vi "RelaySwitcherB2023.vi"(8 "error in (no error)":errorcluster, 10 "RF Position":u16=1 min=1 max=63 step=1, 11 "Device In":cluster{"GPIB":u8, "Address":u8}={"GPIB"=1, "Address"=6} {"Address" min=1 max=31; "GPIB" min=1 max=5}) -> (0 "error out":errorcluster, 1 "concatenated string":string, 3 "Device Out":cluster{"GPIB":u8, "Address":u8}={"GPIB"=1, "Address"=6} {"Address" min=1 max=31; "GPIB" min=1 max=5})   [LabVIEW 2023]
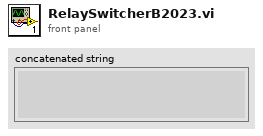
[diagram p1: front panel]
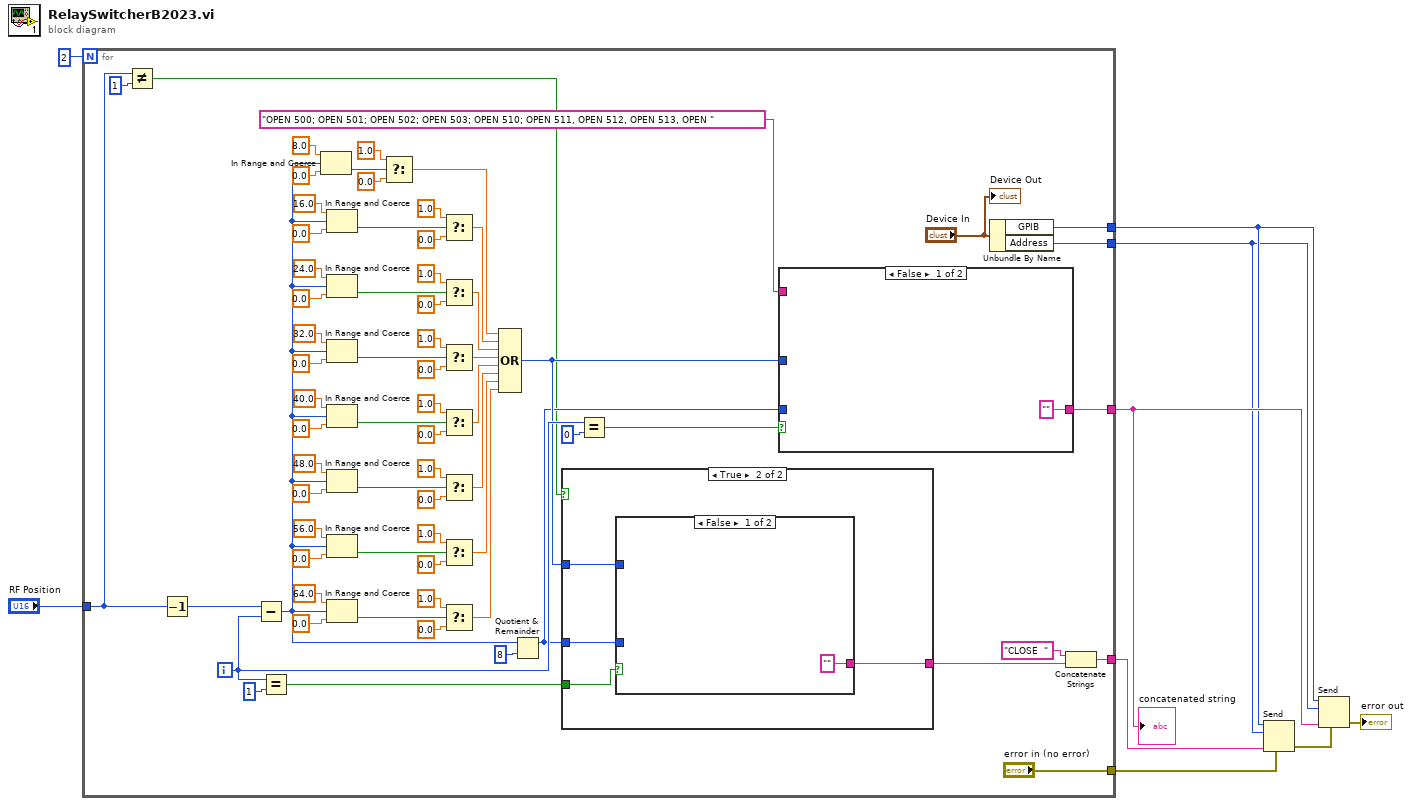
[diagram p0: block diagram]
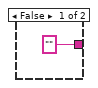
[diagram p2: hidden frame]
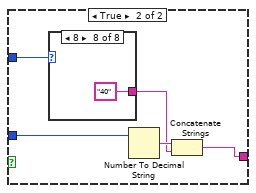
[diagram p3: hidden frame]
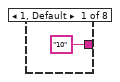
[diagram p4: hidden frame]
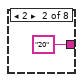
[diagram p5: hidden frame]
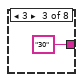
[diagram p6: hidden frame]
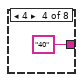
[diagram p7: hidden frame]
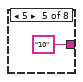
[diagram p8: hidden frame]
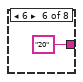
[diagram p9: hidden frame]
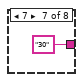
[diagram p10: hidden frame]
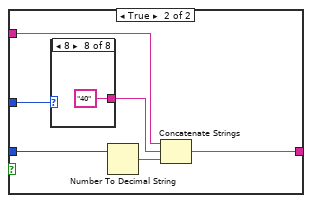
[diagram p11: hidden frame]
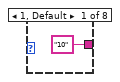
[diagram p12: hidden frame]
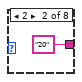
[diagram p13: hidden frame]
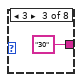
[diagram p14: hidden frame]
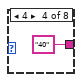
[diagram p15: hidden frame]
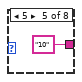
[diagram p16: hidden frame]
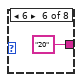
[diagram p17: hidden frame]
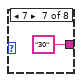
[diagram p18: hidden frame]
diagram:
  n1 = for {
    N: 2 -> [_]
    tunnel: "RF Position" -> [w12]
    tunnel: [w27] -> w5
    tunnel: [w14] -> w4
    tunnel: [w26] -> w3
    tunnel: [w25] -> w2
    tunnel: ["error in (no error)"] -> w1
    i -> [w21]
    n2 = Not Equal?(x=w12, y=u16 1) -> (x != y?=w10:bool)
    n3 = Decrement(x=w12) -> (x-1=w20:u16)
    n4 = Subtract(x=w20, y=w21) -> (x-y=w19:i32)
    n5 = Equal?(x=w21, y=1) -> (x = y?=w13:bool)
    n6 = In Range and Coerce(upper limit=8.0, x=w19, lower limit=0.0) -> (In Range?=w68:bool)  [unwired: 1 out]
    n7 = In Range and Coerce(upper limit=16.0, x=w19, lower limit=0.0) -> (In Range?=w69:bool)  [unwired: 1 out]
    n8 = In Range and Coerce(upper limit=24.0, x=w19, lower limit=0.0) -> (In Range?=w70:bool)  [unwired: 1 out]
    n9 = In Range and Coerce(upper limit=32.0, x=w19, lower limit=0.0) -> (In Range?=w71:bool)  [unwired: 1 out]
    n10 = In Range and Coerce(upper limit=40.0, x=w19, lower limit=0.0) -> (In Range?=w48:bool)  [unwired: 1 out]
    n11 = In Range and Coerce(upper limit=48.0, x=w19, lower limit=0.0) -> (In Range?=w49:bool)  [unwired: 1 out]
    n12 = In Range and Coerce(upper limit=56.0, x=w19, lower limit=0.0) -> (In Range?=w50:bool)  [unwired: 1 out]
    n13 = In Range and Coerce(upper limit=64.0, x=w19, lower limit=0.0) -> (In Range?=w51:bool)  [unwired: 1 out]
    n14 = Select(t=1.0, s=w68, f=0.0) -> (s? t:f=w38:dbl)
    n15 = Select(t=1.0, s=w69, f=0.0) -> (s? t:f=w37:dbl)
    n16 = Select(t=1.0, s=w70, f=0.0) -> (s? t:f=w36:dbl)
    n17 = Select(t=1.0, s=w71, f=0.0) -> (s? t:f=w35:dbl)
    n18 = Select(t=1.0, s=w48, f=0.0) -> (s? t:f=w34:dbl)
    n19 = Select(t=1.0, s=w49, f=0.0) -> (s? t:f=w33:dbl)
    n20 = Select(t=1.0, s=w50, f=0.0) -> (s? t:f=w32:dbl)
    n21 = Select(t=1.0, s=w51, f=0.0) -> (s? t:f=w31:dbl)
    n22 = Compound Arithmetic op=OR(w38, w37, w36, w35, w34, w33, w32, w31) -> (w17:i32)
    n23 = Quotient & Remainder(x=w19, y=u16 8) -> (x-y*floor(x/y)=w15:i32)  [unwired: 1 out]
    n24 = case shown="True" w10 {
      tunnel: w15 -> [_ w84]
      tunnel: ["" w83] -> w18
      tunnel: w17 -> [_ w82]
      tunnel: w13 -> [_ w81]
      frame False {
      }
      frame True {
        n25 = case shown="False" w81 {
          tunnel: w84 -> [_ w90]
          tunnel: ["" w87] -> w83
          tunnel: w82 -> [_ w86]
          frame False {
          }
          frame True {
            n26 = case shown="8" w86 {
              tunnel: ["10" "20" "30" "40" "10" "20" "30" "40"] -> w88
              frame 1, Default {
              }
              frame 2 {
              }
              frame 3 {
              }
              frame 4 {
              }
              frame 5 {
              }
              frame 6 {
              }
              frame 7 {
              }
              frame 8 {
              }
            }
            n27 = Number To Decimal String(number=w90) -> (decimal integer string=w89:string)  [unwired: 1 in]
            n28 = Concatenate Strings(w89, w88) -> (w87:string)
          }
        }
      }
    }
    n29 = Equal?(x=w21, y=0) -> (x = y?=w30:bool)
    n30 = case shown="False" w30 {
      tunnel: w17 -> [_ w105]
      tunnel: "OPEN 500; OPEN 501; OPEN 502; OPEN 503; OPEN 510; OPEN 511, OPEN 512, OPEN 513, OPEN " ("data string") -> [_ w103]
      tunnel: w15 -> [_ w101]
      tunnel: ["" w100] -> w14
      frame False {
      }
      frame True {
        n31 = case shown="8" w105 {
          tunnel: ["10" "20" "30" "40" "10" "20" "30" "40"] -> w102
          frame 1, Default {
          }
          frame 2 {
          }
          frame 3 {
          }
          frame 4 {
          }
          frame 5 {
          }
          frame 6 {
          }
          frame 7 {
          }
          frame 8 {
          }
        }
        n32 = Number To Decimal String(number=w101) -> (decimal integer string=w104:string)  [unwired: 1 in]
        n33 = Concatenate Strings(w103, w102, w104) -> (w100:string)
      }
    }
    n34 = Unbundle By Name("Device In") -> ("GPIB"=w26:u8, "Address"=w25:u8)
    n35 = Concatenate Strings("CLOSE  ", w18) -> (w27:string)
    "Device Out" <- "Device In"
  }
  "concatenated string" <- w4
  n36 = Send(0:w3, 2:w2, 4:w1, 5:w5) -> (8:w9:errorcluster)  [unwired: 1 in, 2 out]
  n37 = Send(0:w3, 2:w2, 4:w9, 5:w4) -> (8:→"error out":errorcluster)  [unwired: 1 in, 2 out]
